vi "Load Configuration File.vi"(10 "advisory dialog? (display:T)":bool=TRUE, 11 "New File Path":path) -> (0 "Files To Acquire":i32, 1 "error":errorcluster, 2 "Data File I/O Information":T1={"Name of Configuration"="", "Path"=path "C:/Users/Achilles/Data/12-20-00", "File Name"="Whole Gel Image", "Files To Acquire"=1, "Current File Number"=21, "Time Limit"=1.0, "Save Data"=FALSE, "Additional Comments"=""}, 3 "new file path":path)   [LabVIEW 2009]
uses:
  Acquisition Settings.vi
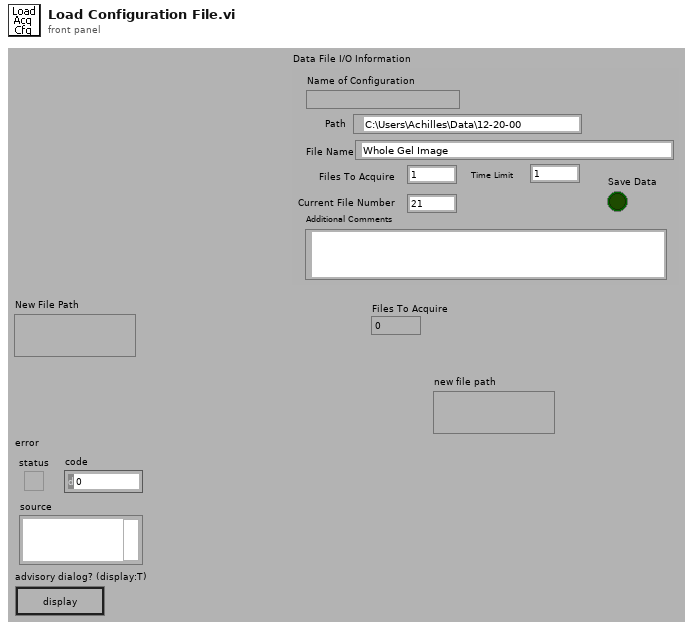
[diagram p1: front panel]
types:
  T1 = cluster{"Name of Configuration":string, "Path":path, "File Name":string, "Files To Acquire":i32, "Current File Number":i32, "Time Limit":dbl, "Save Data":bool, "Additional Comments":string}
  T2 = enum16{"open", "open or create", "create or replace", "create", "open (read only)"}
  T3 = cluster{"Name":string, "Device Number":i16, "Counter Number":i16, "Pulse Spec 1 (Clocks)":u32, "Pulse Spec 2 (Clocks)":u32, "Signal Routing Configuration":i16}[]
  T4 = cluster{"Name":string, "Signal Routing":cluster{"signal name":u16, "signal source":u16, "signal source line number":u32, "signal name line number":u32}[]}[]
  T5 = cluster{"Name":string, "Device Number":i16, "Counter Number":i16, "Line Type for Gate":u32, "Line Number for Gate":u32, "Line Type for Source":u32, "Line Number for Source":u32, "Transfer Method":u32, "Signal Routing Configuration":i16}[]
  T6 = cluster{"Device Number":i16, "Counter Number":i16, "Signal Routing Configuration":i16}
  T7 = cluster{"device":i16, "channel":tag, "buffer size":i32, "Signal Description":cluster{"Name":string, "signal type":enum16{"Sine Wave", "Square Wave", "Sawtooth", "Triangle Wave"}, "period":dbl, "amplitude":dbl, "phase (0 deg)":dbl, "offset (0.0)":dbl, "resting voltage":dbl, "% duty cycle":dbl}[], "clock source (internal:1)":u16, "Clock Line Number":i16}[]
  T8 = cluster{"Device Number":i16, "Counter Number":i16, "Line Type for Source":u32, "Line Number for Source":u32, "Signal Routing Configuration":i16}
  T9 = cluster{"Name":string, "Device Number":i16, "Counter Number":i16, "Pulse Spec 1 (Clocks)":u32, "Pulse Spec 2 (Clocks)":u32, "Signal Routing Configuration":i16, "Inverted":bool}[]
  T10 = cluster{"Name":string, "Device Number":i16, "Counter Number":i16, "Pulse Spec 1 (Clocks)":u32, "Pulse Spec 2 (Clocks)":u32, "Signal Routing Configuration":i16, "Inverted":bool}
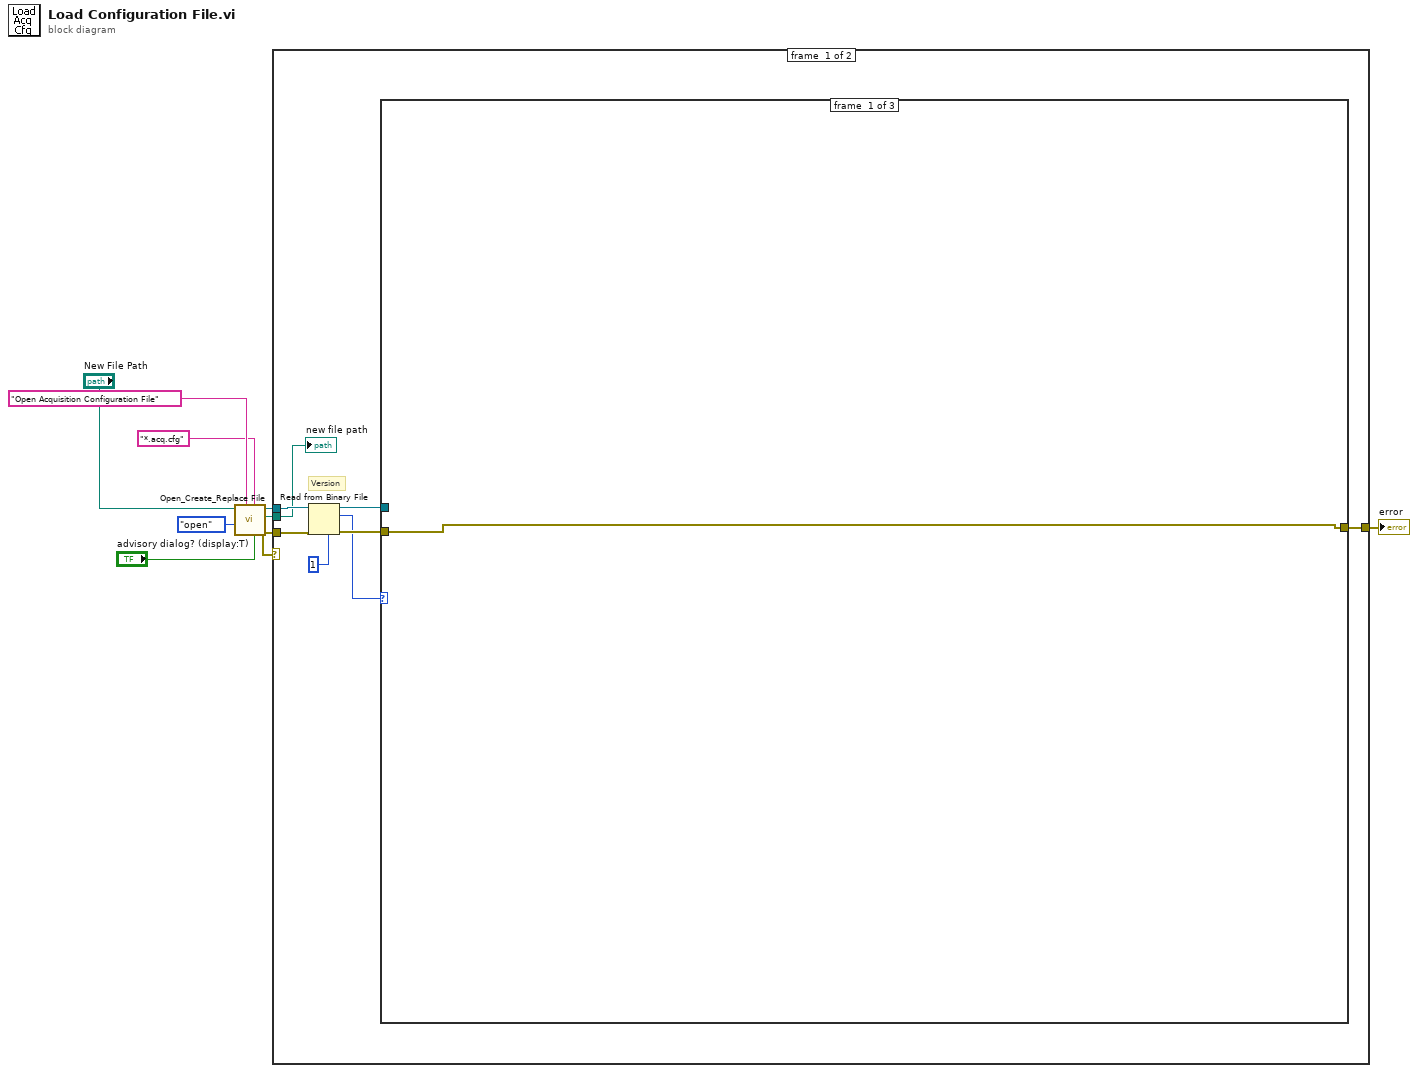
[diagram p0: block diagram]
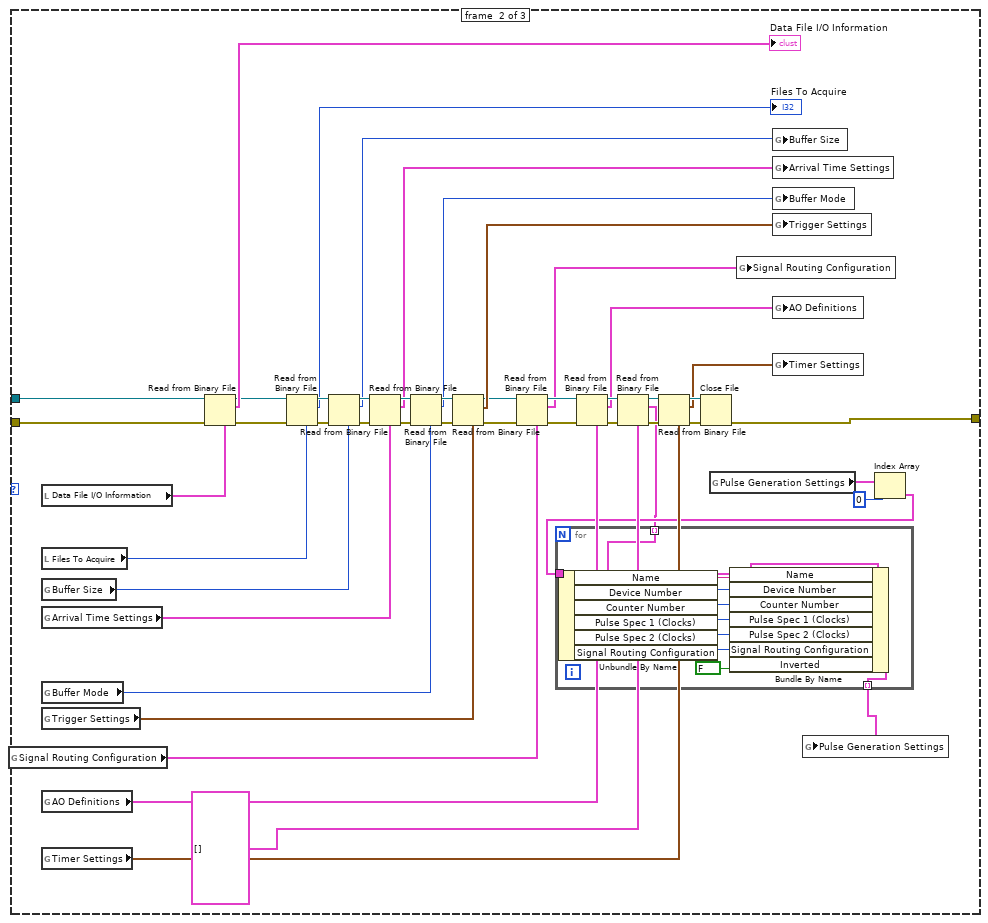
[diagram p2: hidden frame]
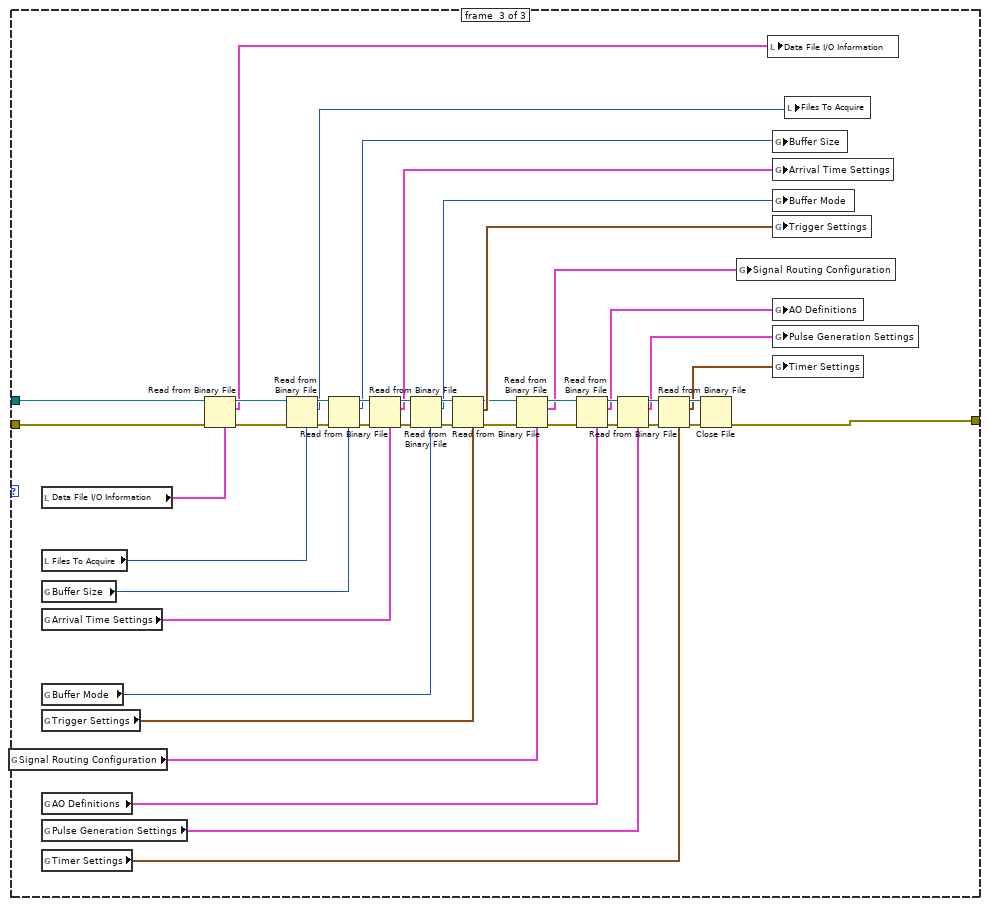
[diagram p3: hidden frame]
diagram:
  n1 = call <vilib>:"Open_Create_Replace File.vi"("advisory dialog? (display:T)"="advisory dialog? (display:T)", "pattern"="*.acq.cfg", "prompt"="Open Acquisition Configuration File", "function (open:0)"=T2."open", "file path"="New File Path") -> ("error out"=w3:errorcluster, "new file path"=w7:path, "refnum"=w8:refnum<file>)  [unwired: 3 in, 1 out]
  n2 = case shown="No Error" w3 {
    selector: w3 -> [_ w119]
    tunnel: w8 -> [w17 _]
    tunnel: w3 -> [w16 _]
    tunnel: w7 -> [w15 _]
    tunnel: [w10 w119] -> w2
    frame #0 {
      # "Version"
      n3 = Read from Binary File(5:1, 8:w16, 11:w17) -> (0:w14:errorcluster, 2:w11:i32, 3:w13:refnum<file>)  [unwired: 3 in, 1 out]
      n4 = case shown="1" w11 {
        tunnel: w14 -> [w18 w65 w118]
        tunnel: w13 -> [_ w64 w117]
        tunnel: [w18 w31 w84] -> w10
        frame #0 {
        }
        frame #1 {
          n5 = global read "Acquisition Settings.vi" "Signal Routing Configuration"() -> (w26:T4)
          n6 = local read "Data File I/O Information"() -> (w49:T1)
          n7 = local read "Files To Acquire"() -> (w48:i32)
          n8 = global read "Acquisition Settings.vi" "Buffer Size"() -> (w47:i32)
          n9 = global read "Acquisition Settings.vi" "Arrival Time Settings"() -> (w46:T5)
          n10 = global read "Acquisition Settings.vi" "Buffer Mode"() -> (w45:u32)
          n11 = global read "Acquisition Settings.vi" "Trigger Settings"() -> (w44:T6)
          n12 = global read "Acquisition Settings.vi" "AO Definitions"() -> (w43:T7)
          n13 = global read "Acquisition Settings.vi" "Timer Settings"() -> (w42:T8)
          n14 = Read from Binary File(5:w49, 8:w65, 11:w64) -> (0:w32:errorcluster, 2:→"Data File I/O Information":T1, 3:w33:refnum<file>)  [unwired: 3 in, 1 out]
          n15 = Read from Binary File(5:w48, 8:w32, 11:w33) -> (0:w63:errorcluster, 2:→"Files To Acquire":i32, 3:w62:refnum<file>)  [unwired: 3 in, 1 out]
          n16 = Read from Binary File(5:w47, 8:w63, 11:w62) -> (0:w61:errorcluster, 2:w39:i32, 3:w60:refnum<file>)  [unwired: 3 in, 1 out]
          n17 = Read from Binary File(5:w46, 8:w61, 11:w60) -> (0:w59:errorcluster, 2:w38:T5, 3:w58:refnum<file>)  [unwired: 3 in, 1 out]
          n18 = Read from Binary File(5:w45, 8:w59, 11:w58) -> (0:w57:errorcluster, 2:w37:u32, 3:w56:refnum<file>)  [unwired: 3 in, 1 out]
          n19 = Read from Binary File(5:w44, 8:w57, 11:w56) -> (0:w29:errorcluster, 2:w36:T6, 3:w30:refnum<file>)  [unwired: 3 in, 1 out]
          n20 = Read from Binary File(5:w26, 8:w29, 11:w30) -> (0:w28:errorcluster, 2:w25:T4, 3:w27:refnum<file>)  [unwired: 3 in, 1 out]
          n21 = Read from Binary File(5:w43, 8:w28, 11:w27) -> (0:w55:errorcluster, 2:w35:T7, 3:w54:refnum<file>)  [unwired: 3 in, 1 out]
          n22 = Read from Binary File(5:T3 [] ("Pulse Generation Settings"), 8:w55, 11:w54) -> (0:w53:errorcluster, 2:w19:T3, 3:w52:refnum<file>)  [unwired: 3 in, 1 out]
          n23 = Read from Binary File(5:w42, 8:w53, 11:w52) -> (0:w51:errorcluster, 2:w34:T8, 3:w50:refnum<file>)  [unwired: 3 in, 1 out]
          n24 = Close File(refnum=w50, error in=w51) -> (error out=w31:errorcluster)  [unwired: 1 out]
          n25 = global read "Acquisition Settings.vi" "Pulse Generation Settings"() -> (w23:T9)
          n26 = global write "Acquisition Settings.vi" "Signal Routing Configuration"(w25) -> ()
          n27 = global write "Acquisition Settings.vi" "Buffer Size"(w39) -> ()
          n28 = global write "Acquisition Settings.vi" "Arrival Time Settings"(w38) -> ()
          n29 = global write "Acquisition Settings.vi" "Buffer Mode"(w37) -> ()
          n30 = global write "Acquisition Settings.vi" "Trigger Settings"(w36) -> ()
          n31 = global write "Acquisition Settings.vi" "AO Definitions"(w35) -> ()
          n32 = global write "Acquisition Settings.vi" "Timer Settings"(w34) -> ()
          n33 = Index Array(array=w23, index=0) -> (element=w21:T10)
          n34 = for {
            tunnel: w21 -> [w75]
            tunnel: [w74] -> w20 mode=indexing
            tunnel: w19 -> [w73] mode=indexing
            n35 = Unbundle By Name(w73) -> ("Name"=w72:string, "Device Number"=w71:i16, "Counter Number"=w70:i16, "Pulse Spec 1 (Clocks)"=w69:u32, "Pulse Spec 2 (Clocks)"=w68:u32, "Signal Routing Configuration"=w67:i16)
            n36 = Bundle By Name(cluster=w75, "Name"=w72, "Device Number"=w71, "Counter Number"=w70, "Pulse Spec 1 (Clocks)"=w69, "Pulse Spec 2 (Clocks)"=w68, "Signal Routing Configuration"=w67, "Inverted"=FALSE) -> (w74:T10)
          }
          n37 = global write "Acquisition Settings.vi" "Pulse Generation Settings"(w20) -> ()
        }
        frame #2 {
          n38 = global read "Acquisition Settings.vi" "Signal Routing Configuration"() -> (w79:T4)
          n39 = local read "Data File I/O Information"() -> (w102:T1)
          n40 = local read "Files To Acquire"() -> (w101:i32)
          n41 = global read "Acquisition Settings.vi" "Buffer Size"() -> (w100:i32)
          n42 = global read "Acquisition Settings.vi" "Arrival Time Settings"() -> (w99:T5)
          n43 = global read "Acquisition Settings.vi" "Buffer Mode"() -> (w98:u32)
          n44 = global read "Acquisition Settings.vi" "Trigger Settings"() -> (w97:T6)
          n45 = global read "Acquisition Settings.vi" "AO Definitions"() -> (w96:T7)
          n46 = global read "Acquisition Settings.vi" "Pulse Generation Settings"() -> (w95:T9)
          n47 = global read "Acquisition Settings.vi" "Timer Settings"() -> (w94:T8)
          n48 = Read from Binary File(5:w102, 8:w118, 11:w117) -> (0:w85:errorcluster, 2:w77:T1, 3:w86:refnum<file>)  [unwired: 3 in, 1 out]
          n49 = Read from Binary File(5:w101, 8:w85, 11:w86) -> (0:w116:errorcluster, 2:w76:i32, 3:w115:refnum<file>)  [unwired: 3 in, 1 out]
          n50 = Read from Binary File(5:w100, 8:w116, 11:w115) -> (0:w114:errorcluster, 2:w93:i32, 3:w113:refnum<file>)  [unwired: 3 in, 1 out]
          n51 = Read from Binary File(5:w99, 8:w114, 11:w113) -> (0:w112:errorcluster, 2:w92:T5, 3:w111:refnum<file>)  [unwired: 3 in, 1 out]
          n52 = Read from Binary File(5:w98, 8:w112, 11:w111) -> (0:w110:errorcluster, 2:w91:u32, 3:w109:refnum<file>)  [unwired: 3 in, 1 out]
          n53 = Read from Binary File(5:w97, 8:w110, 11:w109) -> (0:w82:errorcluster, 2:w90:T6, 3:w83:refnum<file>)  [unwired: 3 in, 1 out]
          n54 = Read from Binary File(5:w79, 8:w82, 11:w83) -> (0:w81:errorcluster, 2:w78:T4, 3:w80:refnum<file>)  [unwired: 3 in, 1 out]
          n55 = Read from Binary File(5:w96, 8:w81, 11:w80) -> (0:w108:errorcluster, 2:w89:T7, 3:w107:refnum<file>)  [unwired: 3 in, 1 out]
          n56 = Read from Binary File(5:w95, 8:w108, 11:w107) -> (0:w106:errorcluster, 2:w88:T9, 3:w105:refnum<file>)  [unwired: 3 in, 1 out]
          n57 = Read from Binary File(5:w94, 8:w106, 11:w105) -> (0:w104:errorcluster, 2:w87:T8, 3:w103:refnum<file>)  [unwired: 3 in, 1 out]
          n58 = Close File(refnum=w103, error in=w104) -> (error out=w84:errorcluster)  [unwired: 1 out]
          n59 = global write "Acquisition Settings.vi" "Signal Routing Configuration"(w78) -> ()
          n60 = local write "Data File I/O Information"(w77) -> ()
          n61 = global write "Acquisition Settings.vi" "Buffer Size"(w93) -> ()
          n62 = global write "Acquisition Settings.vi" "Arrival Time Settings"(w92) -> ()
          n63 = global write "Acquisition Settings.vi" "Buffer Mode"(w91) -> ()
          n64 = global write "Acquisition Settings.vi" "Trigger Settings"(w90) -> ()
          n65 = global write "Acquisition Settings.vi" "AO Definitions"(w89) -> ()
          n66 = global write "Acquisition Settings.vi" "Pulse Generation Settings"(w88) -> ()
          n67 = global write "Acquisition Settings.vi" "Timer Settings"(w87) -> ()
          n68 = local write "Files To Acquire"(w76) -> ()
        }
      }
      "new file path" <- w15
    }
    frame #1 {
    }
  }
  "error" <- w2
